vi "remove zero from 2d array.vi"(6 "page number":i32, 11 "Cycle data by seq":dbl[][](array[numeric])) -> (3 "array w/ subset deleted":dbl[][](array[numeric]))   [LabVIEW 2016]
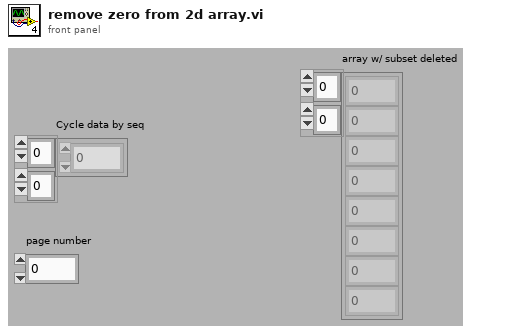
[diagram p1: front panel]
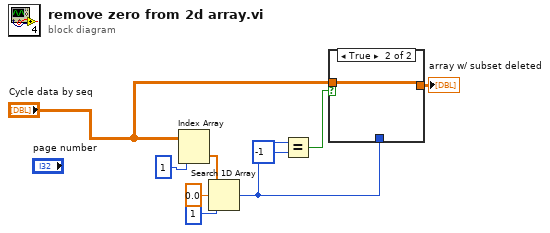
[diagram p0: block diagram]
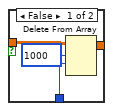
[diagram p2: hidden frame]
diagram:
  n1 = Index Array(array="Cycle data by seq", index (col)=1 ("disabled index (col)")) -> (element=w9:dbl[])  [unwired: 1 in]
  n2 = Search 1D Array(1D array=w9, element=0.0, start index (0)=1) -> (index of element=w3:i32)
  n3 = Equal?(x=w3, y=-1) -> (x = y?=w1:bool)
  n4 = case shown="True" w1 {
    tunnel: [w12 w14] -> w6
    tunnel: "Cycle data by seq" -> [w11 w14]
    tunnel: w3 -> [w10 _]
    frame False {
      n5 = Delete From Array(array=w11, length=1000, index (row)=w10) -> (array with subset deleted=w12:dbl[][])  [unwired: 1 in, 1 out]
    }
    frame True {
    }
  }
  "array w/ subset deleted" <- w6
